vi "Match Tags to CalibEqns.vi"(8 "error in (no error)":errorcluster, 10 "[[APU Calibration Info]]":string[][](array[string]), 11 "Cluster of Arrays":variant) -> (0 "error out":errorcluster, 1 "New Equations":bool, 2 "Found Equation?":bool[](array[boolean]), 3 "Tags and Equations":T1[](array[typedef]))   [LabVIEW 2018, in "RT - Analysis.lvlib"]
doc: "Uses the APU Setup info to match parameters (Indicator Name) with their tags. It outputs all parameters with their value as a 1D array."
uses:
  RT - Analysis.lvlib
  Private Controls/Tag Equation Cluster.ctl
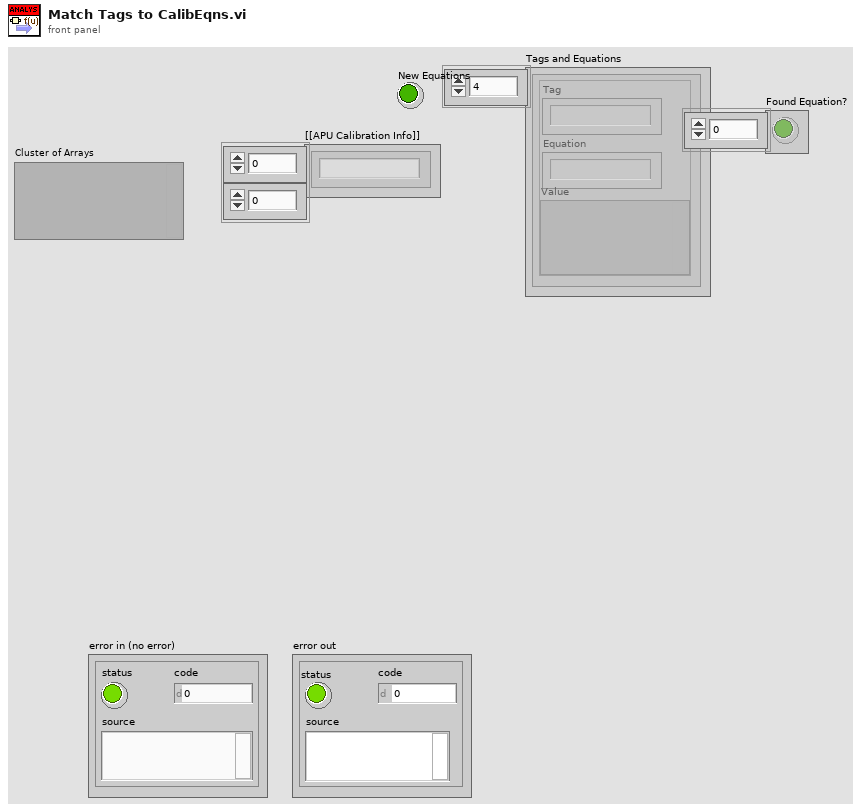
[diagram p1: front panel]
types:
  T1 = typedef "RT - Analysis.lvlib/Tag Equation Cluster.ctl" = cluster{"Tag":string, "Equation":string, "Value":variant}
  T2 = typedef "Parsed Tag Cluster.ctl" = cluster{"Whole Tag":string, "# of Sections":u8, "Chassis":u8, "Slot":u8, "Module":string, "Channel":u8, "SubChannel":u8}
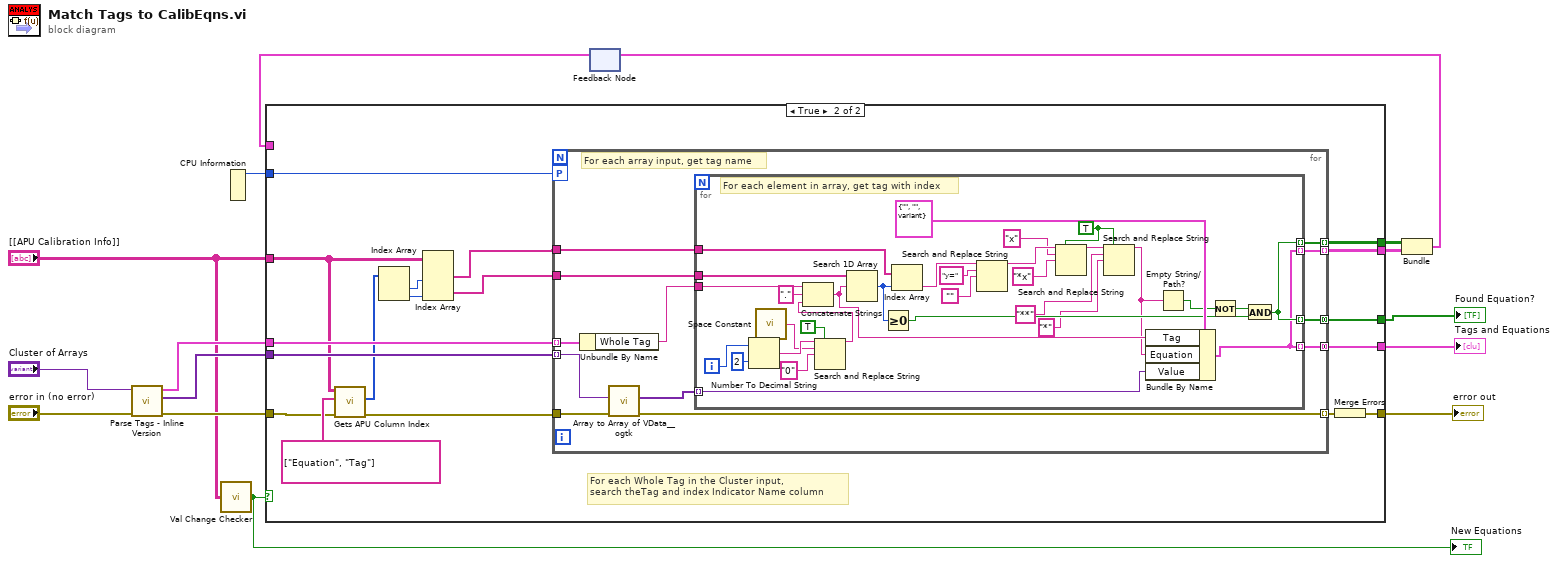
[diagram p0: block diagram]
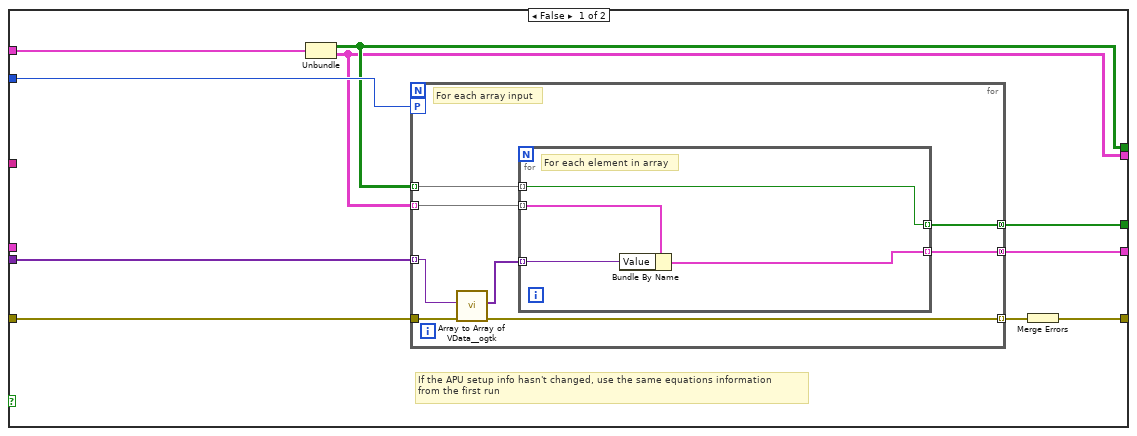
[diagram p2: hidden frame]
diagram:
  n1 = call "Parse Tags - Inline Version.vi"("error in (no error)"="error in (no error)", "Cluster of Controls"="Cluster of Arrays") -> ("error out"=w3:errorcluster, "[VData out]"=w4:variant[], "[Parsed Tags]"=w5:T2[])  [unwired: 6 in, 1 out]
  n2 = call "Val Change Checker.vi"("Current Value in"="[[APU Calibration Info]]") -> ("Value Change?"=w1:bool)
  "New Equations" <- w1
  n3 = CPU Information() -> (4:w12:i32)  [unwired: 3 out]
  n4 = feedback #1() -> (w8:cluster{bool[][], T1[][]})  [unwired: 1 in]
  n5 = case shown="True" w1 {
    tunnel: w4 -> [w23 w55]
    tunnel: w5 -> [_ w54]
    tunnel: [w16 w53] -> w10
    tunnel: w3 -> [w22 w39]
    tunnel: [w20 w51] -> w13
    tunnel: [w17 w50] -> w11
    tunnel: w12 -> [w24 w49]
    tunnel: w8 -> [w25 _]
    tunnel: [w19 w48] -> w7
    tunnel: [w18 w47] -> w6
    tunnel: "[[APU Calibration Info]]" -> [_ w40]
    frame False {
      # "If the APU setup info hasn't changed, use the same equations information\nfrom the first run"
      n6 = Unbundle(w25) -> (w19:bool[][], w18:T1[][])
      n7 = for {
        workers-P: w24 -> [_]
        tunnel: w23 -> [w33] mode=indexing
        tunnel: w22 -> [w32]
        tunnel: [w31] -> w21 mode=indexing
        tunnel: w19 -> [w29] mode=indexing
        tunnel: w18 -> [w28] mode=indexing
        tunnel: [w27] -> w17 mode=concatenating
        tunnel: [w26] -> w16 mode=concatenating
        # "For each array input"
        n8 = call <userlib>:"Array to Array of VData__ogtk.vi"("error in (no error)"=w32, "MultiD Array"=w33) -> ("error out"=w31:errorcluster, "1D Array of Variants"=w30:variant[])  [unwired: 8 in]
        n9 = for {
          tunnel: w30 -> [w35] mode=indexing
          tunnel: w29 -> [w37] mode=indexing
          tunnel: w28 -> [w36] mode=indexing
          tunnel: [w37] -> w27 mode=indexing
          tunnel: [w34] -> w26 mode=indexing
          # "For each element in array"
          n10 = Bundle By Name(cluster=w36, "Value"=w35) -> (w34:T1)
        }
      }
      n11 = Merge Errors(w21) -> (w20:errorcluster)
    }
    frame True {
      # "For each Whole Tag in the Cluster input,\nsearch theTag and index Indicator Name column"
      n12 = call "Gets APU Column Index.vi"("error in (no error)"=w39, "[Column Names]"=string[] ["Equation", "Tag"], "[[Array of Info]]"=w40) -> ("error out"=w38:errorcluster, "[Col Indices]"=w44:i32[])  [unwired: 4 in, 3 out]
      n13 = Index Array(array=w44) -> (element #1=w45:i32, element #2=w46:i32)  [unwired: 2 in]
      n14 = Index Array(array=w40, index (col) #1=w45, index (col) #2=w46) -> (element #1=w42:string[], element #2=w41:string[])  [unwired: 2 in]
      n15 = for {
        tunnel: w54 -> [w67] mode=indexing
        tunnel: w55 -> [w62] mode=indexing
        tunnel: w42 -> [w64]
        tunnel: w41 -> [w66]
        tunnel: [w63] -> w53 mode=concatenating
        tunnel: w38 -> [w61]
        tunnel: [w60] -> w52 mode=indexing
        tunnel: [w58] -> w50 mode=concatenating
        workers-P: w49 -> [_]
        tunnel: [w57] -> w48 mode=indexing
        tunnel: [w56] -> w47 mode=indexing
        # "For each array input, get tag name"
        n16 = Unbundle By Name(w67) -> ("Whole Tag"=w65:string)
        n17 = call <userlib>:"Array to Array of VData__ogtk.vi"("error in (no error)"=w61, "MultiD Array"=w62) -> ("error out"=w60:errorcluster, "1D Array of Variants"=w59:variant[])  [unwired: 8 in]
        n18 = for {
          tunnel: w66 -> [w98]
          tunnel: w65 -> [w91]
          tunnel: w64 -> [w97]
          tunnel: [w79] -> w63 mode=indexing
          tunnel: w59 -> [w83] mode=indexing
          tunnel: [w80] -> w58 mode=indexing
          tunnel: [w80] -> w57 mode=indexing
          tunnel: [w79] -> w56 mode=indexing
          i -> [w96]
          w77 = TRUE ("replace all? (F)")
          # "For each element in array, get tag with index"
          n19 = Number To Decimal String(number=w96, width (-)=i16 2) -> (decimal integer string=w94:string)
          n20 = call <vilib>:"Space Constant.vi"() -> ("String"=w93:string)
          n21 = Search and Replace String(replace all?=TRUE ("replace all? (F)"), input string=w94, search string=w93, replace string="0" ("replace string (\"\")")) -> (result string=w90:string)  [unwired: 4 in, 3 out]
          n22 = Concatenate Strings(w91, "." ("string"), w90) -> (w85:string)
          n23 = Search 1D Array(1D array=w98, element=w85) -> (index of element=w87:i32)  [unwired: 1 in]
          n24 = Greater Or Equal To 0?(x=w87) -> (x >= 0?=w84:bool)
          n25 = Index Array(array=w97, index=w87) -> (element=w69:string)
          n26 = Search and Replace String(input string=w69, search string="y=", replace string="") -> (result string=w75:string)  [unwired: 5 in, 3 out]
          n27 = Search and Replace String(replace all?=w77, input string=w75, search string="x", replace string="*x" ("replace string (\"\")")) -> (result string=w76:string)  [unwired: 4 in, 3 out]
          n28 = Search and Replace String(replace all?=w77, input string=w76, search string="**", replace string="*" ("replace string (\"\")")) -> (result string=w68:string)  [unwired: 4 in, 3 out]
          n29 = Bundle By Name(cluster=T1 {"Tag"="", "Equation"="", "Value"=variant} ("Param Val Cluster"), "Tag"=w85, "Equation"=w68, "Value"=w83) -> (w79:T1)
          n30 = Empty String/Path?(string/path=w68) -> (empty?=w82:bool)
          n31 = Not(x=w82) -> (.not. x?=w81:bool)
          n32 = And(x=w81, y=w84) -> (x .and. y?=w80:bool)
        }
      }
      n33 = Merge Errors(w52) -> (w51:errorcluster)
    }
  }
  "error out" <- w13
  "Tags and Equations" <- w10
  "Found Equation?" <- w11
  n34 = Bundle(w7, w6) -> (w9:cluster{bool[][], T1[][]})  [unwired: 1 in]
  n35 = feedback-in #1(w9) -> ()
